vi "Main.vi"() -> ()   [LabVIEW 2015]
uses:
  TypeDefs/FlowData.ctl
  TypeDefs/FluidData.ctl
  TypeDefs/SetFlow.ctl
  TypeDefs/PDCSetup.ctl
  TypeDefs/PDCDisplay.ctl
  TypeDefs/PDCRecordStatus.ctl
  TypeDefs/PDCFrames.ctl
  TypeDefs/PDCSaveSettings.ctl
  TypeDefs/SetRegulation.ctl
  TypeDefs/AutoTrigger.ctl
  TypeDefs/MPXMicropump.ctl
  TypeDefs/PDCLists.ctl
  TypeDefs/ClsLastSample.ctl
  <vilib>/picture/picture.llb/imagedata.ctl
  <vilib>/Utility/xml.llb/Write to XML File(string).vi
  <vilib>/Utility/xml.llb/Read From XML File(string).vi
panel:
  in  "Run Calibration":bool
  in  "Logging Path":path
  in  "FullDropImpact":bool
  in  "MPX Micropump":T1 {"Signal Form" items=["Sinus", "Rechteck", "SRS-Signal"]}
  out "PDCRecordStatus":T2
  out "Standard Deviation of \nFilm Hight over the \nMeasuring Length [µm]":dbl
  in  "ConfigureCls":bool
  out "Film Height [µm]":dbl
  in  "Set Regulation":T3
  out "SaveStatus":i32(slide)=-2046 caption="Downloading Frames from Camera and Saving.... PLEASE WAIT" scale=-200.0..200.0
  out "Picture":picture
  out "Drop Temperature [°C]":dbl
  out "Angle [°]":dbl format="%#.1g"
  in  "Set Flow":T4 {"Set Flow Value" min=0.0 max=100.0}
  out "Fluid Data":T5
  in  "Log Data":bool
  out "Flow Data":T6
  in  "StopALL":bool
  in  "CamTab":enum32{"CamLIVE", "CamSAVE", "PFV"}(tab)
  in  "PDC Setup":T7={"Color Type"=enum."MONO", "Bit Depth"=0, "Resolution"=0, "Record Rate"=0, "Shutter Speed"=0, "Trigger Mode"=0, "Display"=enum."LiveStop"}
  in  "Record":bool caption="Calibrate"
  in  "RecCancel":bool caption="Calibrate"
  in  "SavePDCSetup":bool
  in  "LoadPDCSetup":bool
  in  "Shading":bool
  in  "Auto Trigger":T9={"Auto Trigger"=FALSE, "Sensitivity [0-100]"=98.4} {"Sensitivity [0-100]" min=0.0 max=100.0 format="%.2f"}
  in  "PDCSaveFrames":bool
  in  "PDC Save Settings":T10={"Save Folder"=path "", "File Name"="", "Data Type"=enum."AVI"}
  in  "PDC Frames":T11 {"Current Frame" min=-39378 max=39378; "End Frame" min=-39378 max=39378; "Start Frame" min=-39378 max=39378; "Frames-Slide" scale=-39378.0..39378.0}
  in  "Path of PFV.exe":path=path "C:/Program Files (x86)/Photron/Photron FASTCAM Viewer 3/PFV.exe"
  in  "PDCStartPFV":bool
  # "Auto Triggering Manual:\n1.) Turn ON 'Auto Trigger' BEFORE pressing 'Record' Button\n2.) Press 'Record' Button and wait 4 sec \n3.) Now ready to recognize Drops automatically."
  # "Run PFV to configure cam/save cam data"
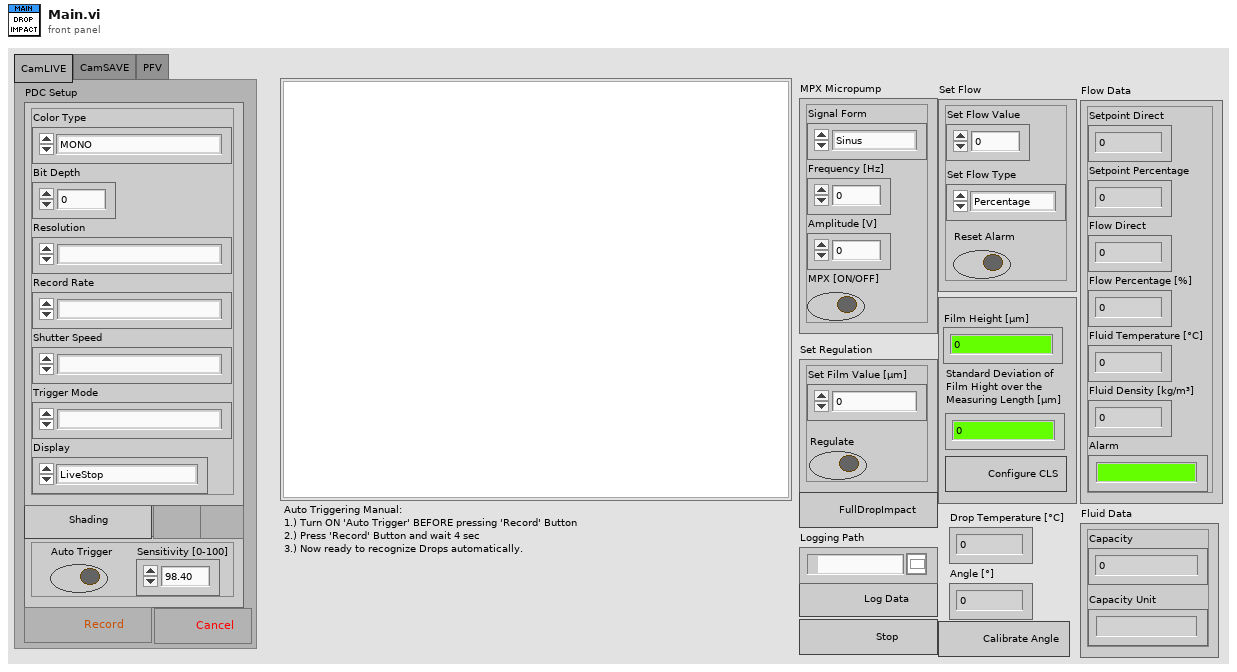
[diagram p1: front panel]
types:
  T1 = typedef "MPXMicropump.ctl" = cluster{"Signal Form":u16, "Frequency [Hz]":i32, "Amplitude [V]":i32, "MPX [ON/OFF]":bool}
  T2 = typedef "PDCRecordStatus.ctl" = enum16{"Live", "Waiting TRG", "Recording"}
  T3 = typedef "SetRegulation.ctl" = cluster{"Set Film Value [µm]":dbl, "Regulate":bool}
  T4 = typedef "SetFlow.ctl" = cluster{"Set Flow Value":dbl, "Set Flow Type":enum16{"Percentage", "Direct"}, "Reset Alarm":bool}
  T5 = typedef "FluidData.ctl" = cluster{"Capacity":sgl, "Capacity Unit":string}
  T6 = typedef "FlowData.ctl" = cluster{"Setpoint Direct":sgl, "Setpoint Percentage":dbl, "Flow Direct":sgl, "Flow Percentage [%]":dbl, "Fluid Temperature [°C]":sgl, "Fluid Density [kg/m³]":sgl, "Alarm":string}
  T7 = typedef "PDCSetup.ctl" = cluster{"Color Type":enum16{"MONO", "COLOR"}, "Bit Depth":i8, "Resolution":u16, "Record Rate":u16, "Shutter Speed":u16, "Trigger Mode":u16, "Display":T8}
  T8 = typedef "PDCDisplay.ctl" = enum16{"Live", "Memory", "LiveStop"}
  T9 = typedef "AutoTrigger.ctl" = cluster{"Auto Trigger":bool, "Sensitivity [0-100]":dbl}
  T10 = typedef "PDCSaveSettings.ctl" = cluster{"Save Folder":path, "File Name":string, "Data Type":enum16{"BMP", "AVI", "MRAW"}}
  T11 = typedef "PDCFrames.ctl" = cluster{"Frames-Slide":i32, "Start Frame":i32, "End Frame":i32, "Current Frame":i32, "PlayFrames":bool}
  T12 = typedef "CommunicationRefs.ctl" = cluster{"ErrorEvent":refnum<user-event>, "DataDisplay":refnum<queue>, "DAQmxAcq":refnum<queue>, "CoriFlow":refnum<queue>, "PrecitecCLS":refnum<queue>, "BartelsMPX":refnum<queue>, "PhotronPDC":refnum<queue>, "JW24F14":refnum<queue>, "Regulator":refnum<queue>, "Logging":refnum<queue>}
  T13 = typedef "ClsLastSample.ctl" = cluster{"Global Signals":dbl[], "Peak Signals":dbl[][], "Film Height [µm]":dbl, "standard deviation [µm]":dbl, "variance":dbl}
  T14 = typedef "PDCLists.ctl" = cluster{"ResolutionList":string[], "RecordRateList":string[], "ShutterSpeedList":string[], "TriggerModeList":string[]}
  T15 = enum8{"Enabled", "Disabled", "Disabled and Grayed Out"}
  T16 = typedef "LVBoundsTypeDef.ctl" = cluster{"Width":u32, "Height":u32}
  T17 = typedef "imagedata.ctl" = cluster{"image type":i32, "image depth":i32, "image":u8[], "mask":u8[], "colors":u32[], "Rectangle":cluster{"left":i16, "top":i16, "right":i16, "bottom":i16}}
  T18 = cluster{"Start":i32, "End":i32, "Trigger":i32, "TwoStageLowToHigh":i32, "TwoStageHighToLow":i32, "TwoStageTiming":u32, "Event":i32[], "EventCount":u32, "RecordedFrames":u32}
  T19 = cluster{"PDC Save Settings":T10, "SaveStatus":refnum<vi>}
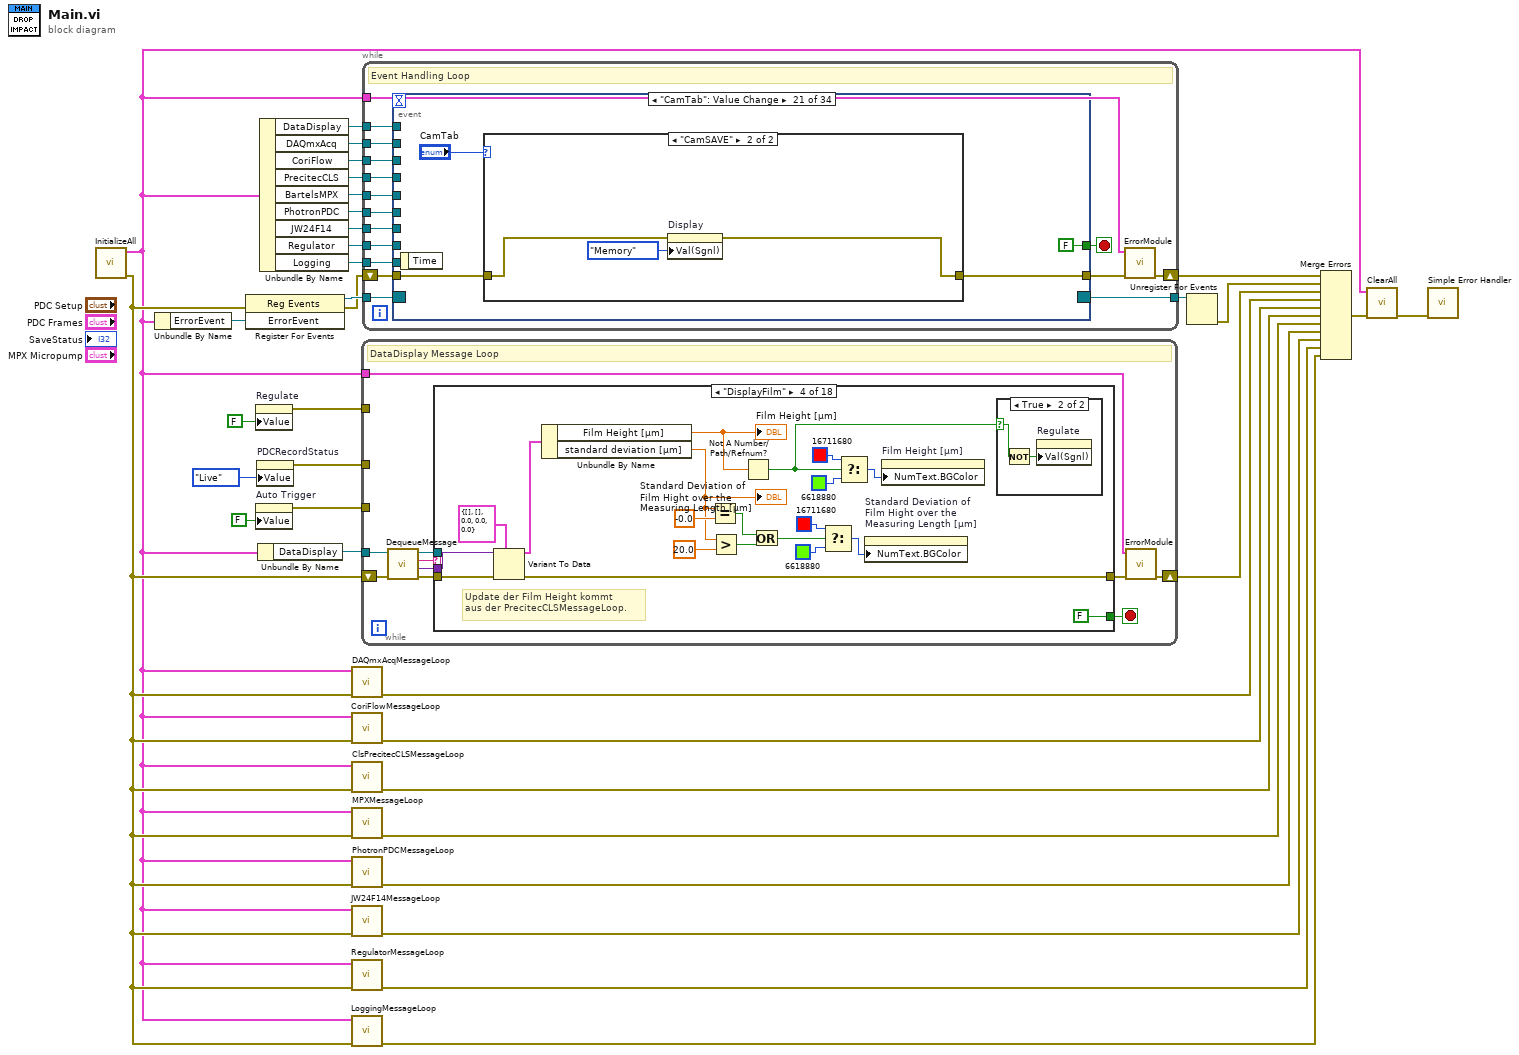
[diagram p0: block diagram]
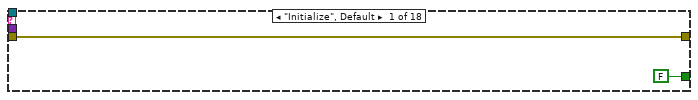
[diagram p2: hidden frame]
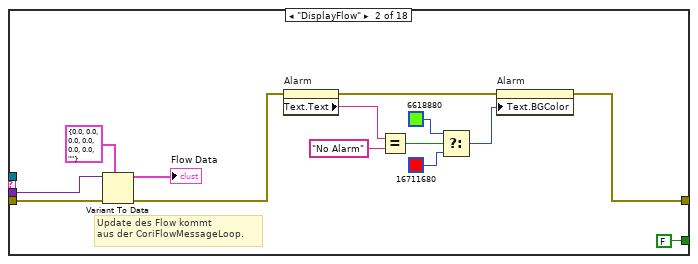
[diagram p3: hidden frame]
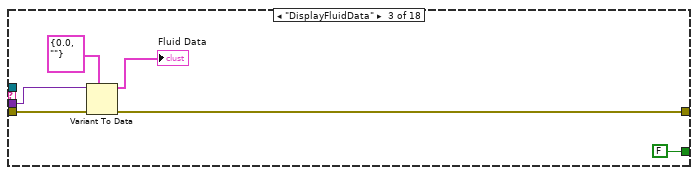
[diagram p4: hidden frame]
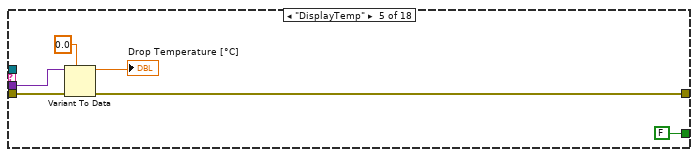
[diagram p6: hidden frame]
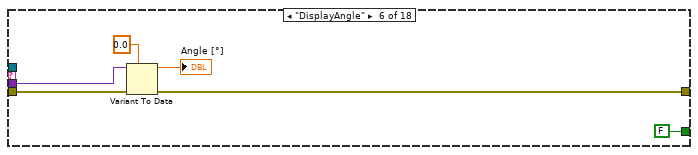
[diagram p7: hidden frame]
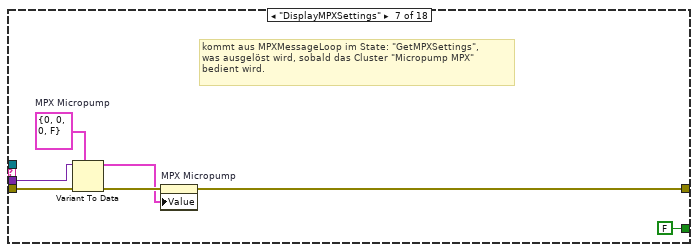
[diagram p8: hidden frame]
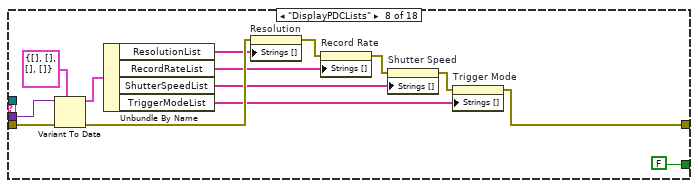
[diagram p9: hidden frame]
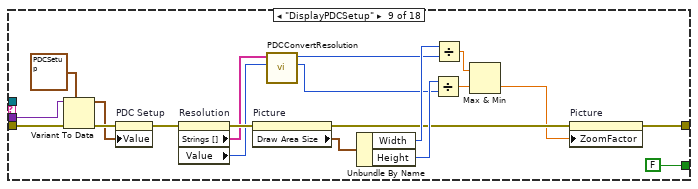
[diagram p10: hidden frame]
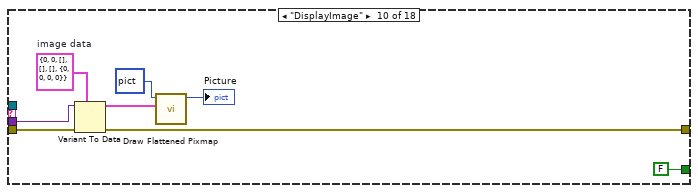
[diagram p11: hidden frame]
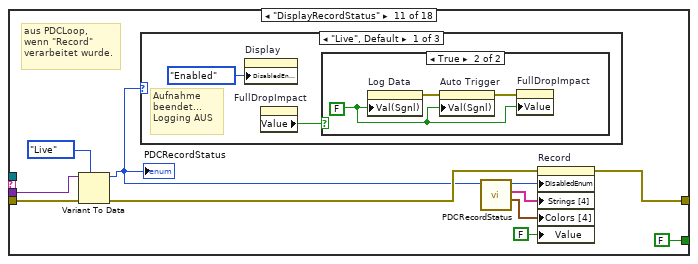
[diagram p12: hidden frame]
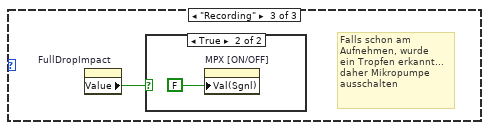
[diagram p15: hidden frame]
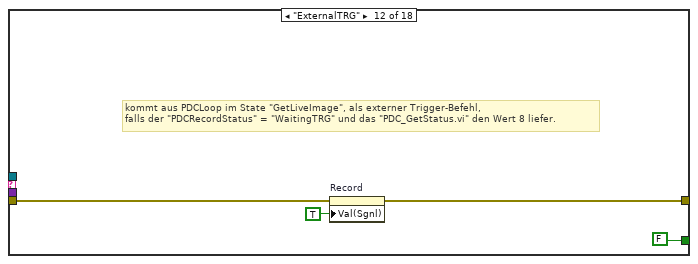
[diagram p17: hidden frame]
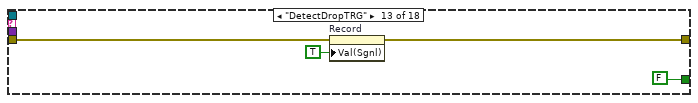
[diagram p18: hidden frame]
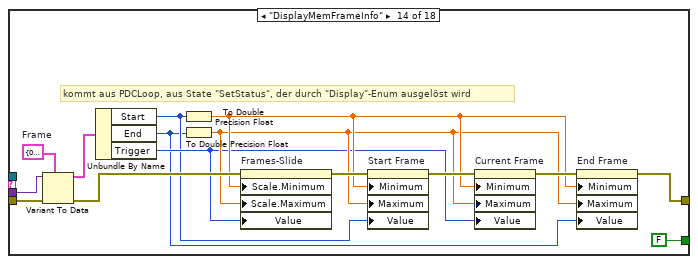
[diagram p19: hidden frame]
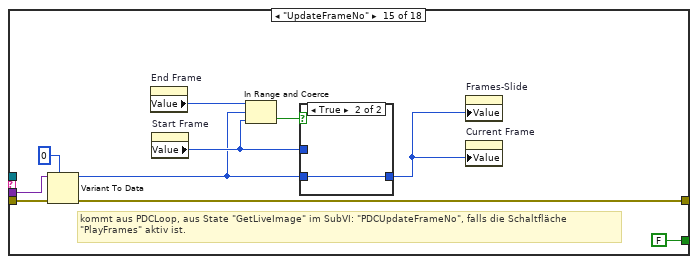
[diagram p20: hidden frame]
diagram:
  n1 = call "InitializeAll.vi"() -> ("Error Out"=w9:errorcluster, "CommunicationRefs"=w1:T12)  [unwired: 10 in]
  n2 = Unbundle By Name(w1) -> ("ErrorEvent"=w30:refnum<user-event>)
  n3 = register-events(error in=w9, w30) -> (reference out=w34:refnum<event-registration>, error out=w31:errorcluster)  [unwired: 1 in]
  n4 = property on="Regulate" class="Bool (strict)"("Value"=FALSE) -> (error out=w2:errorcluster)  [unwired: 2 in, 1 out]
  n5 = property on="Auto Trigger" class="Bool (strict)"("Value"=FALSE) -> (error out=w4:errorcluster)  [unwired: 2 in, 1 out]
  n6 = property on="PDCRecordStatus" class="Enum (strict)"("Value"=PDCRecordStatus."Live" ("PDCRecordStatus")) -> (error out=w12:errorcluster)  [unwired: 2 in, 1 out]
  n7 = Unbundle By Name(w1) -> ("DataDisplay"=w23:refnum<queue>)
  n8 = Unbundle By Name(w1) -> ("DataDisplay"=w21:refnum<queue>, "DAQmxAcq"=w20:refnum<queue>, "CoriFlow"=w19:refnum<queue>, "PrecitecCLS"=w18:refnum<queue>, "BartelsMPX"=w17:refnum<queue>, "PhotronPDC"=w16:refnum<queue>, "JW24F14"=w13:refnum<queue>, "Regulator"=w6:refnum<queue>, "Logging"=w10:refnum<queue>)
  n9 = call "DAQmxAcqMessageLoop.vi"("Error In"=w9, "CommunicationRefs"=w1) -> ("Error Out"=w27:errorcluster)  [unwired: 9 in]
  n10 = call "CoriFlowMessageLoop.vi"("Error In"=w9, "CommunicationRefs"=w1) -> ("Error Out"=w26:errorcluster)  [unwired: 9 in]
  n11 = call "ClsPrecitecCLSMessageLoop.vi"("Error In"=w9, "CommunicationRefs"=w1) -> ("Error Out"=w25:errorcluster)  [unwired: 9 in]
  n12 = call "MPXMessageLoop.vi"("Error In"=w9, "CommunicationRefs"=w1) -> ("Error Out"=w24:errorcluster)  [unwired: 9 in]
  n13 = call "PhotronPDCMessageLoop.vi"("Error In"=w9, "CommunicationRefs"=w1) -> ("Error Out"=w15:errorcluster)  [unwired: 9 in]
  n14 = call "JW24F14MessageLoop.vi"("Error In"=w9, "CommunicationRefs"=w1) -> ("Error Out"=w14:errorcluster)  [unwired: 9 in]
  n15 = call "RegulatorMessageLoop.vi"("Error In"=w9, "CommunicationRefs"=w1) -> ("Error Out"=w8:errorcluster)  [unwired: 9 in]
  n16 = call "LoggingMessageLoop.vi"("Error In"=w9, "CommunicationRefs"=w1) -> ("Error Out"=w7:errorcluster)  [unwired: 9 in]
  n17 = while {
    tunnel: w23 -> [w45]
    tunnel: w1 -> [w38]
    shift-right: [w39] -> w22
    shift-left: w9 -> [w44]
    tunnel: w12 -> [_]
    tunnel: w4 -> [_]
    tunnel: w2 -> [_]
    stop <- w37 stop-if-true
    # "DataDisplay Message Loop"
    n18 = call "DequeueMessage.vi"("error in (no error)"=w44, "MessageQueue"=w45) -> ("error out"=w40:errorcluster, "MessageData"=w41:variant, "Message"=w42:string, "dupMessageQueue"=w43:refnum<queue>)  [unwired: 6 in]
    n19 = case shown="\"DisplayFilm\"" w42 {
      tunnel: w43 -> [_ _ _ _ _ _ _ _ _ _ _ _ _ _ _ _ _ _]
      tunnel: w41 -> [_ w61 w65 w85 w94 w99 w107 w120 w140 w148 w158 _ _ w190 w199 _ _ _]
      tunnel: w40 -> [w46 w60 w67 w86 w91 w98 w108 w121 w142 w150 w160 w172 w174 w191 w200 w206 w210 w219]
      tunnel: [w46 w49 w66 w76 w90 w97 w104 w109 w129 w147 w151 w171 w173 w182 w197 w204 w208 w219] -> w36
      tunnel: [FALSE FALSE FALSE FALSE FALSE FALSE FALSE FALSE FALSE FALSE FALSE FALSE FALSE FALSE FALSE FALSE FALSE TRUE] -> w37
      frame "Initialize", Default {
      }
      frame "DisplayFlow" {
        # "Update des Flow kommt \naus der CoriFlowMessageLoop."
        n20 = Variant To Data(error in=w60, type=T6 {"Setpoint Direct"=0.0, "Setpoint Percentage"=0.0, "Flow Direct"=0.0, "Flow Percentage [%]"=0.0, "Fluid Temperature [°C]"=0.0, "Fluid Density [kg/m³]"=0.0, "Alarm"=""} ("Sensor Data"), Variant=w61) -> (data=→"Flow Data":T6, error out=w52:errorcluster)
        n21 = property on="Alarm" class="Str"(error in=w52) -> (error out=w50:errorcluster, "Text.Text"=w51:string)  [unwired: 1 in, 1 out]
        n22 = Equal?(x=w51, y="No Alarm") -> (x = y?=w56:bool)
        n23 = Select(t=u32 6618880, s=w56, f=u32 16711680) -> (s? t:f=w48:u32)
        n24 = property on="Alarm" class="Str"(error in=w50, "Text.BGColor"=w48) -> (error out=w49:errorcluster)  [unwired: 1 in, 1 out]
      }
      frame "DisplayFluidData" {
        n25 = Variant To Data(error in=w67, type=T5 {"Capacity"=0.0, "Capacity Unit"=""} ("Fluid Data"), Variant=w65) -> (data=→"Fluid Data":T5, error out=w66:errorcluster)
      }
      frame "DisplayFilm" {
        # "Update der Film Height kommt \naus der PrecitecCLSMessageLoop."
        n26 = Variant To Data(error in=w86, type=T13 {"Global Signals"=[], "Peak Signals"=[], "Film Height [µm]"=0.0, "standard deviation [µm]"=0.0, "variance"=0.0} ("ClsLastSample"), Variant=w85) -> (data=w83:T13, error out=w76:errorcluster)
        n27 = Unbundle By Name(w83) -> ("Film Height [µm]"=w82:dbl, "standard deviation [µm]"=w78:dbl)
        "Film Height [µm]" <- w82
        "Standard Deviation of \nFilm Hight over the \nMeasuring Length [µm]" <- w78
        n28 = Equal?(x=w78, y=-0.0) -> (x = y?=w80:bool)
        n29 = Greater?(x=w78, y=20.0) -> (0:w79:bool)
        n30 = Not A Number/Path/Refnum?(number/path/refnum=w82) -> (NaN/Path/Refnum?=w68:bool)
        n31 = Or(x=w80, y=w79) -> (x .or. y?=w73:bool)
        n32 = Select(t=u32 16711680, s=w73, f=u32 6618880) -> (s? t:f=w72:u32)
        n33 = Select(t=u32 16711680, s=w68, f=u32 6618880) -> (s? t:f=w69:u32)
        n34 = property on="Standard Deviation of \nFilm Hight over the \nMeasuring Length [µm]" class="DigNum (strict)"("NumText.BGColor"=w72) -> ()  [unwired: 2 in, 2 out]
        n35 = property on="Film Height [µm]" class="DigNum (strict)"("NumText.BGColor"=w69) -> ()  [unwired: 2 in, 2 out]
        n36 = case shown="True" w68 {
          selector: w68 -> [_ w89]
          frame False {
          }
          frame True {
            n37 = Not(x=w89) -> (.not. x?=w88:bool)
            n38 = property on="Regulate" class="Bool (strict)"("Val(Sgnl)"=w88) -> ()  [unwired: 2 in, 2 out]
          }
        }
      }
      frame "DisplayTemp" {
        n39 = Variant To Data(error in=w91, type=0.0, Variant=w94) -> (data=→"Drop Temperature [°C]":dbl, error out=w90:errorcluster)
      }
      frame "DisplayAngle" {
        n40 = Variant To Data(error in=w98, type=0.0, Variant=w99) -> (data=→"Angle [°]":dbl, error out=w97:errorcluster)
      }
      frame "DisplayMPXSettings" {
        w103 = T1 {"Signal Form"=0, "Frequency [Hz]"=0, "Amplitude [V]"=0, "MPX [ON/OFF]"=FALSE}  # MPX Micropump
        # "kommt aus MPXMessageLoop im State: \"GetMPXSettings\",\nwas ausgelöst wird, sobald das Cluster \"Micropump MPX\"\nbedient wird."
        n41 = Variant To Data(error in=w108, type=w103, Variant=w107) -> (data=w102:T1, error out=w105:errorcluster)
        n42 = property on="MPX Micropump" class="Clust (strict)"(error in=w105, "Value"=w102) -> (error out=w104:errorcluster)  [unwired: 1 in, 1 out]
      }
      frame "DisplayPDCLists" {
        n43 = Variant To Data(error in=w121, type=T14 {"ResolutionList"=[], "RecordRateList"=[], "ShutterSpeedList"=[], "TriggerModeList"=[]} ("PDCLists"), Variant=w120) -> (data=w117:T14, error out=w122:errorcluster)
        n44 = Unbundle By Name(w117) -> ("ResolutionList"=w116:string[], "RecordRateList"=w115:string[], "ShutterSpeedList"=w113:string[], "TriggerModeList"=w110:string[])
        n45 = property on="Resolution" class="Ring (strict)"(error in=w122, "Strings []"=w116) -> (error out=w114:errorcluster)  [unwired: 1 in, 1 out]
        n46 = property on="Record Rate" class="Ring (strict)"(error in=w114, "Strings []"=w115) -> (error out=w112:errorcluster)  [unwired: 1 in, 1 out]
        n47 = property on="Shutter Speed" class="Ring (strict)"(error in=w112, "Strings []"=w113) -> (error out=w111:errorcluster)  [unwired: 1 in, 1 out]
        n48 = property on="Trigger Mode" class="Ring (strict)"(error in=w111, "Strings []"=w110) -> (error out=w109:errorcluster)  [unwired: 1 in, 1 out]
      }
      frame "DisplayPDCSetup" {
        n49 = Variant To Data(error in=w142, type=T7 {"Color Type"=enum."MONO", "Bit Depth"=0, "Resolution"=0, "Record Rate"=0, "Shutter Speed"=0, "Trigger Mode"=0, "Display"=enum."LiveStop"} ("PDC Setup"), Variant=w140) -> (data=w137:T7, error out=w138:errorcluster)
        n50 = property on="PDC Setup" class="Clust (strict)"(error in=w138, "Value"=w137) -> (error out=w132:errorcluster)  [unwired: 1 in, 1 out]
        n51 = property on="Resolution" class="Ring (strict)"(error in=w132) -> (error out=w131:errorcluster, "Strings []"=w127:string[], "Value"=w126:u16)  [unwired: 1 in, 1 out]
        n52 = property on="Picture" class="Pict"(error in=w131) -> (error out=w128:errorcluster, "Draw Area Size"=w130:T16)  [unwired: 1 in, 1 out]
        n53 = call "PDCConvertResolution.vi"("ResValue"=w126, "ResStrings"=w127) -> ("Height"=w124:u32, "Width"=w125:u32)  [unwired: 8 in]
        n54 = Unbundle By Name(w130) -> ("Width"=w133:u32, "Height"=w134:u32)
        n55 = Divide(x=w134, y=w124) -> (x/y=w136:dbl)
        n56 = Divide(x=w133, y=w125) -> (x/y=w135:dbl)
        n57 = Max & Min(x=w135, y=w136) -> (min(x,y)=w123:dbl)  [unwired: 1 out]
        n58 = property on="Picture" class="Pict"(error in=w128, "ZoomFactor"=w123) -> (error out=w129:errorcluster)  [unwired: 1 in, 1 out]
      }
      frame "DisplayImage" {
        w146 = T17 {"image type"=0, "image depth"=0, "image"=[], "mask"=[], "colors"=[], "Rectangle"={"left"=0, "top"=0, "right"=0, "bottom"=0}}  # image data
        n59 = Variant To Data(error in=w150, type=w146, Variant=w148) -> (data=w145:T17, error out=w147:errorcluster)
        n60 = call <vilib>:"Draw Flattened Pixmap.vi"("image data"=w145, "picture"=picture data[5B]) -> ("new picture"=→"Picture":picture)  [unwired: 7 in]
      }
      frame "DisplayRecordStatus" {
        # "aus PDCLoop, \nwenn \"Record\" \nverarbeitet wurde."
        n61 = Variant To Data(error in=w160, type=PDCRecordStatus."Live" ("PDCRecordStatus"), Variant=w158) -> (data=w152:T2, error out=w161:errorcluster)
        "PDCRecordStatus" <- w152
        n62 = case shown="\"Live\", Default" w152 {
          frame "Live", Default {
            # "Aufnahme\nbeendet...\nLogging AUS"
            n63 = property on="Display" class="Enum (strict)"("DisabledEnum"=T15."Enabled" ("Disabled")) -> ()  [unwired: 2 in, 2 out]
            n64 = property on="FullDropImpact" class="Bool (strict)"() -> ("Value"=w162:bool)  [unwired: 2 in, 2 out]
            n65 = case shown="True" w162 {
              frame False {
              }
              frame True {
                w164 = FALSE ("Value (Signaling)")
                n66 = property on="Log Data" class="Bool (strict)"("Val(Sgnl)"=w164) -> (error out=w166:errorcluster)  [unwired: 2 in, 1 out]
                n67 = property on="Auto Trigger" class="Bool (strict)"(error in=w166, "Val(Sgnl)"=w164) -> (error out=w165:errorcluster)  [unwired: 1 in, 1 out]
                n68 = property on="FullDropImpact" class="Bool (strict)"(error in=w165, "Value"=w164) -> ()  [unwired: 1 in, 2 out]
              }
            }
          }
          frame "Waiting TRG" {
          }
          frame "Recording" {
            # "Falls schon am \nAufnehmen, wurde\nein Tropfen erkannt...\ndaher Mikropumpe \nausschalten"
            n69 = property on="FullDropImpact" class="Bool (strict)"() -> ("Value"=w167:bool)  [unwired: 2 in, 2 out]
            n70 = case shown="True" w167 {
              frame False {
              }
              frame True {
                n71 = property on="MPX [ON/OFF]" class="Bool (strict)"("Val(Sgnl)"=FALSE ("Value (Signaling)")) -> ()  [unwired: 2 in, 2 out]
              }
            }
          }
        }
        n72 = call "PDCRecordStatus.vi"("PDCRecordStatus"=w152) -> ("Color[4]"=w154:cluster{u32, u32}[], "String[4]"=w156:string[], "Disabled"=w155:T15)  [unwired: 8 in]
        n73 = property on="Record" class="Bool (strict)"(error in=w161, "DisabledEnum"=w155, "Strings [4]"=w156, "Colors [4]"=w154, "Value"=FALSE ("Record")) -> (error out=w151:errorcluster)  [unwired: 1 in, 1 out]
      }
      frame "ExternalTRG" {
        # "kommt aus PDCLoop im State \"GetLiveImage\", als externer Trigger-Befehl,\nfalls der \"PDCRecordStatus\" = \"WaitingTRG\" und das \"PDC_GetStatus.vi\" den Wert 8 liefer."
        n74 = property on="Record" class="Bool (strict)"(error in=w172, "Val(Sgnl)"=TRUE ("Value (Signaling)")) -> (error out=w171:errorcluster)  [unwired: 1 in, 1 out]
      }
      frame "DetectDropTRG" {
        n75 = property on="Record" class="Bool (strict)"(error in=w174, "Val(Sgnl)"=TRUE ("Value (Signaling)")) -> (error out=w173:errorcluster)  [unwired: 1 in, 1 out]
      }
      frame "DisplayMemFrameInfo" {
        w189 = T18 {"Start"=0, "End"=0, "Trigger"=0, "TwoStageLowToHigh"=0, "TwoStageHighToLow"=0, "TwoStageTiming"=0, "Event"=[1, 1, 1, 1, 1, 1, 1, 1, 1, 1], "EventCount"=0, "RecordedFrames"=0}  # Frame
        # "kommt aus PDCLoop, aus State \"SetStatus\", der durch \"Display\"-Enum ausgelöst wird"
        n76 = Variant To Data(error in=w191, type=w189, Variant=w190) -> (data=w188:T18, error out=w186:errorcluster)
        n77 = Unbundle By Name(w188) -> ("Start"=w178:i32, "End"=w177:i32, "Trigger"=w179:i32)
        n78 = To Double Precision Float(number=w178) -> (double precision float=w181:dbl)
        n79 = To Double Precision Float(number=w177) -> (double precision float=w180:dbl)
        n80 = property on="Frames-Slide" class="Slide (strict)"(error in=w186, "Scale.Minimum"=w181, "Scale.Maximum"=w180, "Value"=w179) -> (error out=w185:errorcluster)  [unwired: 1 in, 1 out]
        n81 = property on="Start Frame" class="DigNum (strict)"(error in=w185, "Minimum"=w181, "Maximum"=w180, "Value"=w178) -> (error out=w184:errorcluster)  [unwired: 1 in, 1 out]
        n82 = property on="Current Frame" class="DigNum (strict)"(error in=w184, "Minimum"=w181, "Maximum"=w180, "Value"=w179) -> (error out=w183:errorcluster)  [unwired: 1 in, 1 out]
        n83 = property on="End Frame" class="DigNum (strict)"(error in=w183, "Minimum"=w181, "Maximum"=w180, "Value"=w177) -> (error out=w182:errorcluster)  [unwired: 1 in, 1 out]
      }
      frame "UpdateFrameNo" {
        # "kommt aus PDCLoop, aus State \"GetLiveImage\" im SubVI: \"PDCUpdateFrameNo\", falls die Schaltfläche\n\"PlayFrames\" aktiv ist."
        n84 = Variant To Data(error in=w200, type=0 ("Value (Signaling)"), Variant=w199) -> (data=w192:i32, error out=w197:errorcluster)
        n85 = property on="End Frame" class="DigNum (strict)"() -> ("Value"=w193:i32)  [unwired: 2 in, 2 out]
        n86 = property on="Start Frame" class="DigNum (strict)"() -> ("Value"=w195:i32)  [unwired: 2 in, 2 out]
        n87 = In Range and Coerce(upper limit=w193, x=w192, lower limit=w195) -> (In Range?=w194:bool)  [unwired: 1 out]
        n88 = case shown="True" w194 {
          tunnel: w195 -> [w202 _]
          tunnel: w192 -> [_ w203]
          tunnel: [w202 w203] -> w196
          frame False {
          }
          frame True {
          }
        }
        n89 = property on="Frames-Slide" class="Slide (strict)"("Value"=w196) -> ()  [unwired: 2 in, 2 out]
        n90 = property on="Current Frame" class="DigNum (strict)"("Value"=w196) -> ()  [unwired: 2 in, 2 out]
      }
      frame "PDCDataSaveFinished" {
        # "kommt aus PDCLoop, aus State \"PDCDataSave\", wenn das Abspeichern der Frames abgeschlossen ist."
        n91 = property on="CamTab" class="TabCtl (strict)"(error in=w206, "DisabledEnum"=T15."Enabled" ("Disabled")) -> (error out=w204:errorcluster)  [unwired: 1 in, 1 out]
      }
      frame "RefImageTaken" {
        n92 = property on="FullDropImpact" class="Bool (strict)"(error in=w210) -> (error out=w209:errorcluster, "Value"=w211:bool)  [unwired: 1 in, 1 out]
        n93 = case shown="True" w211 {
          tunnel: w209 -> [w213 w215]
          tunnel: [w213 w214] -> w208
          frame False {
          }
          frame True {
            w216 = TRUE ("Value (Signaling)")
            n94 = property on="MPX [ON/OFF]" class="Bool (strict)"(error in=w215, "Val(Sgnl)"=w216) -> (error out=w217:errorcluster)  [unwired: 1 in, 1 out]
            n95 = property on="Log Data" class="Bool (strict)"(error in=w217, "Val(Sgnl)"=w216) -> (error out=w214:errorcluster)  [unwired: 1 in, 1 out]
          }
        }
      }
      frame "Stop" {
      }
    }
    n96 = call "ErrorModule.vi"("Error In"=w36, "CommunicationRefs"=w38) -> ("Error Out"=w39:errorcluster)  [unwired: 9 in]
  }
  n97 = while {
    tunnel: w34 -> [w235]
    tunnel: [w233] -> w33
    shift-right: [w231] -> w29
    shift-left: w31 -> [w232]
    tunnel: w1 -> [w229]
    tunnel: w20 -> [w228]
    tunnel: w19 -> [w227]
    tunnel: w18 -> [w226]
    tunnel: w17 -> [w225]
    tunnel: w6 -> [w224]
    tunnel: w21 -> [w223]
    tunnel: w16 -> [w222]
    tunnel: w13 -> [w221]
    tunnel: w10 -> [w220]
    stop <- w234 stop-if-true
    # "Event Handling Loop"
    n98 = event shown="[20] \"CamTab\": Value Change" {
      selector: w235 -> [_ _ _ _ _ _ _ _ _ _ _ _ _ _ _ _ _ _ _ _ _ _ _ _ _ _ _ _ _ _ _ _ _ _]
      dyn-events: [_ _ _ _ _ _ _ _ _ _ _ _ _ _ _ _ _ _ _ _ _ _ _ _ _ _ _ _ _ _ _ _ _ _] -> w233
      timeout: _ -> [_ _ _ _ _ _ _ _ _ _ _ _ _ _ _ _ _ _ _ _ _ _ _ _ _ _ _ _ _ _ _ _ _ _]
      tunnel: ["StopALL" w252 FALSE ("Error") FALSE ("Error") FALSE ("Error") FALSE ("Error") FALSE ("Error") FALSE ("Error") FALSE ("Error") FALSE ("Error") FALSE ("Error") FALSE ("Error") FALSE ("Error") FALSE ("Error") FALSE ("Error") FALSE ("Error") FALSE ("Error") FALSE ("Error") FALSE ("Error") FALSE ("Error") FALSE ("Error") FALSE ("Error") FALSE ("Error") FALSE ("Error") FALSE ("Error") FALSE ("Error") FALSE ("Error") FALSE ("Error") FALSE ("Error") FALSE ("Error") FALSE ("Error") FALSE ("Error") FALSE ("Error") FALSE ("Error")] -> w234
      tunnel: [w247 w251 w263 w288 w301 w306 w313 w337 w344 w351 w358 w365 w372 w375 w393 w402 w405 w414 w429 w432 w441 w452 w459 w483 w507 w522 w532 w552 w568 w592 w598 w615 w646 w681] -> w230
      tunnel: w232 -> [w247 w251 w264 w284 w302 w307 w314 w338 w345 w352 w359 w366 w373 w376 w394 w403 w412 w419 w423 w436 w442 w455 w456 w480 w513 w523 w524 w553 w570 w593 w599 w616 w645 w682]
      tunnel: w228 -> [w245 _ w261 _ _ _ _ _ _ _ _ _ _ _ _ _ _ _ _ _ _ _ _ _ _ _ _ _ _ _ _ _ _ _]
      tunnel: w227 -> [w244 _ w260 w293 w303 _ _ _ _ _ _ _ _ _ _ _ _ _ _ _ _ _ _ _ _ _ _ _ _ _ _ _ _ _]
      tunnel: w226 -> [w243 _ w259 _ _ _ _ _ _ _ _ _ _ _ _ _ _ _ _ _ _ _ _ _ _ _ _ _ _ _ _ _ _ w684]
      tunnel: w225 -> [w242 _ w258 _ _ _ _ w339 w346 w353 w360 _ _ _ _ _ _ _ _ _ _ _ _ _ _ _ _ _ _ _ _ _ _ _]
      tunnel: w224 -> [w237 _ _ _ _ w311 _ _ _ _ _ _ _ _ _ _ _ _ _ _ _ _ _ _ _ _ _ _ _ _ _ _ _ _]
      tunnel: w223 -> [w241 _ _ _ _ _ _ _ _ _ _ _ _ _ _ _ _ _ _ _ _ _ _ _ _ _ _ _ _ _ _ _ _ _]
      tunnel: w222 -> [w239 _ w255 _ _ _ _ _ _ _ _ w367 w374 w386 w395 w404 w413 w420 w428 w438 _ _ w457 w481 w506 w520 w530 _ w567 w590 w596 w611 _ _]
      tunnel: w221 -> [w238 _ w254 _ _ _ _ _ _ _ _ _ _ _ _ _ _ _ _ _ _ _ _ _ _ _ _ _ _ _ _ _ w644 _]
      tunnel: w220 -> [w236 _ w253 _ _ _ _ _ _ _ _ _ _ _ _ _ _ _ _ _ _ _ _ _ _ _ _ _ _ _ _ _ _ _]
      event "StopALL": Value Change; Panel Close {
        # "Stoppt die Event-Schleife und sendet eine Nachricht \nan alle anderen Schleifen zum Stoppen."
        n99 = event-data() -> ()  [unwired: 1 in, 1 out]
        n100 = Build Array(w241, w245, w244, w243, w242, w239, w238, w237, w236) -> (w240:refnum<queue>[])
        n101 = for {
          tunnel: w240 -> [w250] mode=indexing
          workers-P: _ -> [_]
          n102 = call "EnqueueMessage.vi"("Priority Message? (F)"=TRUE, "Message"="Stop", "MessageQueue"=w250) -> ()  [unwired: 7 in, 2 out]
        }
      }
      event User Event {
        # "Das ErrorEvent wird ausgelöst, falls in einer der Schleifen ein Error\ndurch das Error-Modul festgestellt wird... und dient zum\nStoppen der Event-Schleife"
        n103 = event-data() -> ("Error"=w252:bool)  [unwired: 1 in]
      }
      event "Log Data": Value Change {
        n104 = event-data() -> ()  [unwired: 1 in, 1 out]
        n105 = Build Array(w261, w260, w259, w258, w255, w254, w253) -> (w257:refnum<queue>[])
        n106 = for {
          tunnel: "Log Data" -> [w266]
          shift-right: [w267] -> w263
          shift-left: w264 -> [w268]
          tunnel: w257 -> [w265] mode=indexing
          n107 = case shown="True" w266 {
            tunnel: w265 -> [w275 w280]
            tunnel: w268 -> [w273 w278]
            tunnel: [w272 w277] -> w267
            frame True {
              n108 = To Variant(anything="Logging Path") -> (Variant=w269:variant)
              n109 = call "EnqueueMessage.vi"("Priority Message? (F)"=TRUE, "error in (no error)"=w273, "MessageData"=w269, "Message"="StartLogging", "MessageQueue"=w275) -> ("error out"=w272:errorcluster)  [unwired: 5 in, 1 out]
            }
            frame False {
              n110 = call "EnqueueMessage.vi"("Priority Message? (F)"=TRUE, "error in (no error)"=w278, "Message"="StopLogging", "MessageQueue"=w280) -> ("error out"=w277:errorcluster)  [unwired: 6 in, 1 out]
            }
          }
        }
      }
      event Value Change {
        n111 = event-data() -> ()  [unwired: 1 in, 1 out]
        n112 = property on="Set Flow Type" class="Enum (strict)"(error in=w284) -> (error out=w283:errorcluster, "Value"=w287:enum16{"Percentage", "Direct"})  [unwired: 1 in, 1 out]
        n113 = case shown="\"Percentage\", Default" w287 {
          tunnel: [sgl 100.0 ("Value") w298] -> w286
          tunnel: w283 -> [w294 w297]
          tunnel: [w294 w296] -> w282
          frame "Percentage", Default {
          }
          frame "Direct" {
            n114 = property on="Capacity" class="DigNum (strict)"(error in=w297) -> (error out=w296:errorcluster, "Value"=w298:sgl)  [unwired: 1 in, 1 out]
          }
        }
        n115 = property on="Set Flow Value" class="DigNum (strict)"(error in=w282, "Maximum"=w286, "Minimum"=0.0 ("Data Entry Limits:Minimum")) -> (error out=w281:errorcluster)  [unwired: 1 in, 1 out]
        n116 = To Variant(anything="Set Flow") -> (Variant=w291:variant)
        n117 = call "EnqueueMessage.vi"("error in (no error)"=w281, "MessageData"=w291, "Message"="SetFlow", "MessageQueue"=w293) -> ("error out"=w288:errorcluster)  [unwired: 6 in, 1 out]
      }
      event Value Change {
        n118 = event-data() -> ()  [unwired: 1 in, 1 out]
        n119 = call "EnqueueMessage.vi"("error in (no error)"=w302, "Message"="ResetAlarm", "MessageQueue"=w303) -> ("error out"=w301:errorcluster)  [unwired: 7 in, 1 out]
      }
      event Value Change {
        n120 = event-data() -> ()  [unwired: 1 in, 1 out]
        n121 = To Variant(anything="Set Regulation") -> (Variant=w310:variant)
        n122 = call "EnqueueMessage.vi"("Priority Message? (F)"=TRUE, "error in (no error)"=w307, "MessageData"=w310, "Message"="SetRegulation", "MessageQueue"=w311) -> ("error out"=w306:errorcluster)  [unwired: 5 in, 1 out]
      }
      event "FullDropImpact": Value Change {
        n123 = event-data() -> ()  [unwired: 1 in, 1 out]
        n124 = case shown="True" "FullDropImpact" {
          tunnel: w314 -> [w316 w319]
          tunnel: [w316 w321] -> w313
          frame False {
          }
          frame True {
            n125 = call "File Dialog3"("pattern (all files)"="*.tdms") -> ("selected path"=w318:path)  [unwired: 11 in, 3 out]
            n126 = call <vilib>:"Is Path and Not Empty.vi"("path"=w318) -> ("Is Path and Not Empty?"=w317:bool)  [unwired: 4 in]
            n127 = case shown="True" w317 {
              tunnel: [w324 w330] -> w321
              tunnel: w318 -> [_ w327]
              tunnel: w319 -> [w324 w326]
              frame False {
                n128 = property on="FullDropImpact" class="Bool (strict)"("Value"=FALSE ("FullDropImpact")) -> ()  [unwired: 2 in, 2 out]
                n129 = One Button Dialog(message="INVALID \"Logging Path\".") -> ()  [unwired: 1 in, 1 out]
              }
              frame True {
                w331 = TRUE ("Value (Signaling)")
                n130 = property on="Logging Path" class="Path"(error in=w326, "Value"=w327) -> (error out=w325:errorcluster)  [unwired: 1 in, 1 out]
                n131 = property on="Regulate" class="Bool (strict)"(error in=w325, "Val(Sgnl)"=FALSE ("Value (Signaling)")) -> (error out=w329:errorcluster)  [unwired: 1 in, 1 out]
                n132 = property on="Auto Trigger" class="Bool (strict)"(error in=w329, "Val(Sgnl)"=w331) -> (error out=w332:errorcluster)  [unwired: 1 in, 1 out]
                n133 = property on="Record" class="Bool (strict)"(error in=w332, "Val(Sgnl)"=w331) -> (error out=w330:errorcluster)  [unwired: 1 in, 1 out]
              }
            }
          }
        }
      }
      event Value Change {
        n134 = event-data() -> ("NewVal"=w333:bool)  [unwired: 1 in]
        n135 = To Variant(anything=w333) -> (Variant=w334:variant)
        n136 = call "EnqueueMessage.vi"("error in (no error)"=w338, "MessageData"=w334, "Message"="SetOnOff", "MessageQueue"=w339) -> ("error out"=w337:errorcluster)  [unwired: 6 in, 1 out]
      }
      event Value Change {
        n137 = event-data() -> ("NewVal"=w340:u16)  [unwired: 1 in]
        n138 = To Variant(anything=w340) -> (Variant=w341:variant)
        n139 = call "EnqueueMessage.vi"("error in (no error)"=w345, "MessageData"=w341, "Message"="SetSignalForm", "MessageQueue"=w346) -> ("error out"=w344:errorcluster)  [unwired: 6 in, 1 out]
      }
      event Value Change {
        n140 = event-data() -> ("NewVal"=w347:i32)  [unwired: 1 in]
        n141 = To Variant(anything=w347) -> (Variant=w348:variant)
        n142 = call "EnqueueMessage.vi"("error in (no error)"=w352, "MessageData"=w348, "Message"="SetFrequency", "MessageQueue"=w353) -> ("error out"=w351:errorcluster)  [unwired: 6 in, 1 out]
      }
      event Value Change {
        n143 = event-data() -> ("NewVal"=w354:i32)  [unwired: 1 in]
        n144 = To Variant(anything=w354) -> (Variant=w355:variant)
        n145 = call "EnqueueMessage.vi"("error in (no error)"=w359, "MessageData"=w355, "Message"="SetAmplitude", "MessageQueue"=w360) -> ("error out"=w358:errorcluster)  [unwired: 6 in, 1 out]
      }
      event Value Change {
        n146 = event-data() -> ("NewVal"=w361:enum16{"MONO", "COLOR"})  [unwired: 1 in]
        n147 = To Variant(anything=w361) -> (Variant=w362:variant)
        n148 = call "EnqueueMessage.vi"("error in (no error)"=w366, "MessageData"=w362, "Message"="SetColorType", "MessageQueue"=w367) -> ("error out"=w365:errorcluster)  [unwired: 6 in, 1 out]
      }
      event Value Change {
        n149 = event-data() -> ("NewVal"=w368:i8)  [unwired: 1 in]
        n150 = To Variant(anything=w368) -> (Variant=w369:variant)
        n151 = call "EnqueueMessage.vi"("error in (no error)"=w373, "MessageData"=w369, "Message"="SetBitDepth", "MessageQueue"=w374) -> ("error out"=w372:errorcluster)  [unwired: 6 in, 1 out]
      }
      event Value Change {
        w377 = cluster{"Width":u32, "Height":u32} {"Width"=0, "Height"=0}  # Resolution
        n152 = event-data() -> ("NewVal"=w381:u16)  [unwired: 1 in]
        n153 = property on="Resolution" class="Ring (strict)"() -> ("Strings []"=w382:string[])  [unwired: 2 in, 2 out]
        n154 = call "PDCConvertResolution.vi"("ResValue"=w381, "ResStrings"=w382) -> ("Height"=w378:u32, "Width"=w379:u32)  [unwired: 8 in]
        n155 = Bundle By Name(cluster=w377, "Width"=w379, "Height"=w378) -> (w380:cluster{"Width":u32, "Height":u32})
        n156 = To Variant(anything=w380) -> (Variant=w383:variant)
        n157 = call "EnqueueMessage.vi"("error in (no error)"=w376, "MessageData"=w383, "Message"="SetResolution", "MessageQueue"=w386) -> ("error out"=w375:errorcluster)  [unwired: 6 in, 1 out]
      }
      event Value Change {
        n158 = event-data() -> ("NewVal"=w388:u16)  [unwired: 1 in]
        n159 = property on="Record Rate" class="Ring (strict)"() -> ("Strings []"=w389:string[])  [unwired: 2 in, 2 out]
        n160 = call "PDCConvertRecRate.vi"("RecRateValue"=w388, "RecRateList"=w389) -> ("RecRate"=w387:u32)  [unwired: 9 in]
        n161 = To Variant(anything=w387) -> (Variant=w390:variant)
        n162 = call "EnqueueMessage.vi"("error in (no error)"=w394, "MessageData"=w390, "Message"="SetRecordRate", "MessageQueue"=w395) -> ("error out"=w393:errorcluster)  [unwired: 6 in, 1 out]
      }
      event Value Change {
        n163 = event-data() -> ("NewVal"=w397:u16)  [unwired: 1 in]
        n164 = property on="Shutter Speed" class="Ring (strict)"() -> ("Strings []"=w398:string[])  [unwired: 2 in, 2 out]
        n165 = call "PDCConvertShutter.vi"("ShutterValue"=w397, "ShutterList"=w398) -> ("ShutterSpeed"=w396:u32)  [unwired: 9 in]
        n166 = To Variant(anything=w396) -> (Variant=w399:variant)
        n167 = call "EnqueueMessage.vi"("error in (no error)"=w403, "MessageData"=w399, "Message"="SetShutterSpeed", "MessageQueue"=w404) -> ("error out"=w402:errorcluster)  [unwired: 6 in, 1 out]
      }
      event Value Change {
        n168 = event-data() -> ("NewVal"=w407:u16)  [unwired: 1 in]
        n169 = property on="Trigger Mode" class="Ring (strict)"() -> ("Strings []"=w408:string[])  [unwired: 2 in, 2 out]
        n170 = call "PDCConvertTrigg.vi"("TriggerValue"=w407, "TriggerStrings"=w408) -> ("TriggerMode"=w406:u32)  [unwired: 9 in]
        n171 = To Variant(anything=w406) -> (Variant=w409:variant)
        n172 = call "EnqueueMessage.vi"("error in (no error)"=w412, "MessageData"=w409, "Message"="SetTriggerMode", "MessageQueue"=w413) -> ("error out"=w405:errorcluster)  [unwired: 6 in, 1 out]
      }
      event Value Change {
        n173 = event-data() -> ("NewVal"=w415:T8)  [unwired: 1 in]
        n174 = To Variant(anything=w415) -> (Variant=w416:variant)
        n175 = call "EnqueueMessage.vi"("error in (no error)"=w419, "MessageData"=w416, "Message"="SetStatus", "MessageQueue"=w420) -> ("error out"=w414:errorcluster)  [unwired: 6 in, 1 out]
      }
      event "Record": Value Change {
        n176 = event-data() -> ()  [unwired: 1 in, 1 out]
        n177 = property on="Display" class="Enum (strict)"(error in=w423, "DisabledEnum"=T15."Disabled and Grayed Out" ("Disabled")) -> (error out=w422:errorcluster)  [unwired: 1 in, 1 out]
        n178 = property on="PDCRecordStatus" class="Enum (strict)"(error in=w422) -> (error out=w426:errorcluster, "Value"=w424:T2)  [unwired: 1 in, 1 out]
        n179 = To Variant(anything=w424) -> (Variant=w425:variant)
        n180 = call "EnqueueMessage.vi"("error in (no error)"=w426, "MessageData"=w425, "Message"="Record", "MessageQueue"=w428) -> ("error out"=w429:errorcluster)  [unwired: 6 in, 1 out]
      }
      event "RecCancel": Value Change {
        n181 = event-data() -> ()  [unwired: 1 in, 1 out]
        n182 = property on="Display" class="Enum (strict)"(error in=w436, "DisabledEnum"=T15."Enabled" ("Disabled")) -> (error out=w434:errorcluster)  [unwired: 1 in, 1 out]
        n183 = call "EnqueueMessage.vi"("error in (no error)"=w434, "Message"="RecStop", "MessageQueue"=w438) -> ("error out"=w433:errorcluster)  [unwired: 7 in, 1 out]
        n184 = property on="RecCancel" class="Bool (strict)"(error in=w433, "Value"=FALSE ("RecCancel")) -> (error out=w432:errorcluster)  [unwired: 1 in, 1 out]
      }
      event "CamTab": Value Change {
        n185 = event-data() -> ()  [unwired: 1 in, 1 out]
        n186 = case shown="\"CamSAVE\"" "CamTab" {
          tunnel: w442 -> [w445 w451]
          tunnel: [w447 w449] -> w441
          frame "CamLIVE", Default {
            n187 = property on="PlayFrames" class="Bool (strict)"(error in=w445, "Value"=FALSE ("CamPlay")) -> (error out=w446:errorcluster)  [unwired: 1 in, 1 out]
            n188 = property on="Display" class="Enum (strict)"(error in=w446, "Val(Sgnl)"=PDCDisplay."Live" ("Value (Signaling)")) -> (error out=w447:errorcluster)  [unwired: 1 in, 1 out]
          }
          frame "CamSAVE" {
            n189 = property on="Display" class="Enum (strict)"(error in=w451, "Val(Sgnl)"=PDCDisplay."Memory" ("Value (Signaling)")) -> (error out=w449:errorcluster)  [unwired: 1 in, 1 out]
          }
        }
      }
      event Value Change {
        n190 = event-data() -> ("NewVal"=w453:i32)  [unwired: 1 in]
        n191 = property on="Current Frame" class="DigNum (strict)"(error in=w455, "Val(Sgnl)"=w453) -> (error out=w452:errorcluster)  [unwired: 1 in, 1 out]
      }
      event Value Change {
        n192 = event-data() -> ("OldVal"=w458:i32, "NewVal"=w460:i32)  [unwired: 1 in]
        n193 = property on="End Frame" class="DigNum (strict)"() -> ("Value"=w462:i32)  [unwired: 2 in, 2 out]
        n194 = Less?(x=w460, y=w462) -> (x < y?=w461:bool)
        n195 = case shown="True" w461 {
          tunnel: w460 -> [_ w466]
          tunnel: [w465 w474] -> w459
          tunnel: w456 -> [w465 w471]
          tunnel: w458 -> [w464 _]
          tunnel: w457 -> [_ w469]
          frame False {
            n196 = property on="Start Frame" class="DigNum (strict)"("Value"=w464) -> ()  [unwired: 2 in, 2 out]
          }
          frame True {
            n197 = To Variant(anything=w466) -> (Variant=w467:variant)
            n198 = call "EnqueueMessage.vi"("error in (no error)"=w471, "MessageData"=w467, "Message"="UpdateStartFrame", "MessageQueue"=w469) -> ("error out"=w470:errorcluster)  [unwired: 6 in, 1 out]
            n199 = property on="Frames-Slide" class="Slide (strict)"() -> ("Value"=w478:i32)  [unwired: 2 in, 2 out]
            n200 = Greater?(x=w466, y=w478) -> (0:w479:bool)
            n201 = Select(t=w466, s=w479, f=w478) -> (s? t:f=w477:i32)
            n202 = property on="Frames-Slide" class="Slide (strict)"("Scale.Minimum"=w466, "Value"=w477) -> (error out=w476:errorcluster)  [unwired: 2 in, 1 out]
            n203 = property on="Current Frame" class="DigNum (strict)"(error in=w470, "Val(Sgnl)"=w477) -> (error out=w475:errorcluster)  [unwired: 1 in, 1 out]
            n204 = Merge Errors(w476, w475) -> (w473:errorcluster)
            n205 = property on="PlayFrames" class="Bool (strict)"(error in=w473, "Val(Sgnl)"=FALSE ("Value (Signaling)")) -> (error out=w474:errorcluster)  [unwired: 1 in, 1 out]
          }
        }
      }
      event Value Change {
        n206 = event-data() -> ("OldVal"=w482:i32, "NewVal"=w484:i32)  [unwired: 1 in]
        n207 = property on="Start Frame" class="DigNum (strict)"() -> ("Value"=w486:i32)  [unwired: 2 in, 2 out]
        n208 = Greater?(x=w484, y=w486) -> (0:w485:bool)
        n209 = case shown="True" w485 {
          tunnel: w484 -> [_ w490]
          tunnel: [w489 w498] -> w483
          tunnel: w480 -> [w489 w495]
          tunnel: w482 -> [w488 _]
          tunnel: w481 -> [_ w493]
          frame False {
            n210 = property on="End Frame" class="DigNum (strict)"("Value"=w488) -> ()  [unwired: 2 in, 2 out]
          }
          frame True {
            n211 = To Variant(anything=w490) -> (Variant=w491:variant)
            n212 = call "EnqueueMessage.vi"("error in (no error)"=w495, "MessageData"=w491, "Message"="UpdateEndFrame", "MessageQueue"=w493) -> ("error out"=w494:errorcluster)  [unwired: 6 in, 1 out]
            n213 = property on="Frames-Slide" class="Slide (strict)"() -> ("Value"=w502:i32)  [unwired: 2 in, 2 out]
            n214 = Less?(x=w490, y=w502) -> (x < y?=w503:bool)
            n215 = Select(t=w490, s=w503, f=w502) -> (s? t:f=w501:i32)
            n216 = property on="Frames-Slide" class="Slide (strict)"("Scale.Maximum"=w490, "Value"=w501) -> (error out=w500:errorcluster)  [unwired: 2 in, 1 out]
            n217 = property on="Current Frame" class="DigNum (strict)"(error in=w494, "Val(Sgnl)"=w501) -> (error out=w499:errorcluster)  [unwired: 1 in, 1 out]
            n218 = Merge Errors(w500, w499) -> (w497:errorcluster)
            n219 = property on="PlayFrames" class="Bool (strict)"(error in=w497, "Val(Sgnl)"=FALSE ("Value (Signaling)")) -> (error out=w498:errorcluster)  [unwired: 1 in, 1 out]
          }
        }
      }
      event Value Change {
        n220 = event-data() -> ("NewVal"=w505:i32)  [unwired: 1 in]
        n221 = property on="End Frame" class="DigNum (strict)"() -> ("Value"=w510:i32)  [unwired: 2 in, 2 out]
        n222 = property on="Start Frame" class="DigNum (strict)"() -> ("Value"=w508:i32)  [unwired: 2 in, 2 out]
        n223 = In Range and Coerce(upper limit=w510, x=w505, lower limit=w508) -> (In Range?=w509:bool)  [unwired: 1 out]
        n224 = case shown="True" w509 {
          tunnel: w508 -> [w515 _]
          tunnel: w505 -> [_ w516]
          tunnel: [w515 w516] -> w504
          frame False {
          }
          frame True {
          }
        }
        n225 = property on="Frames-Slide" class="Slide (strict)"("Value"=w504) -> ()  [unwired: 2 in, 2 out]
        n226 = property on="Current Frame" class="DigNum (strict)"("Value"=w504) -> ()  [unwired: 2 in, 2 out]
        n227 = To Variant(anything=w504) -> (Variant=w511:variant)
        n228 = call "EnqueueMessage.vi"("error in (no error)"=w513, "MessageData"=w511, "Message"="UpdateCurrentFrame", "MessageQueue"=w506) -> ("error out"=w507:errorcluster)  [unwired: 6 in, 1 out]
      }
      event Value Change {
        n229 = event-data() -> ("NewVal"=w517:bool)  [unwired: 1 in]
        n230 = To Variant(anything=w517) -> (Variant=w519:variant)
        n231 = call "EnqueueMessage.vi"("error in (no error)"=w523, "MessageData"=w519, "Message"="TogglePlayFrames", "MessageQueue"=w520) -> ("error out"=w522:errorcluster)  [unwired: 6 in, 1 out]
      }
      event "PDCSaveFrames": Value Change {
        n232 = event-data() -> ()  [unwired: 1 in, 1 out]
        n233 = Unbundle By Name("PDC Save Settings") -> ("Save Folder"=w528:path, "File Name"=w527:string)
        n234 = Build Path(base path=w528, name or relative path=w527) -> (appended path=w526:path)
        n235 = Empty String/Path?(string/path=w526) -> (empty?=w525:bool)
        n236 = case shown="False" w525 {
          tunnel: w524 -> [w533 w544]
          tunnel: [w541 w544] -> w532
          tunnel: w530 -> [w540 _]
          tunnel: "PDC Save Settings" -> [w536 _]
          frame False {
            n237 = control-ref of="SaveStatus"() -> (w542:refnum<vi>)
            n238 = property on="CamTab" class="TabCtl (strict)"(error in=w533, "DisabledEnum"=2) -> (error out=w534:errorcluster)  [unwired: 1 in, 1 out]
            n239 = Bundle("PDC Save Settings"=w536, "SaveStatus"=w542) -> (w538:T19)  [unwired: 1 in]
            n240 = To Variant(anything=w538) -> (Variant=w539:variant)
            n241 = call "EnqueueMessage.vi"("error in (no error)"=w534, "MessageData"=w539, "Message"="PDCDataSave", "MessageQueue"=w540) -> ("error out"=w541:errorcluster)  [unwired: 6 in, 1 out]
          }
          frame True {
            n242 = One Button Dialog(message="File Name ERROR.\nPlease check \"Save Folder\"/\"File Name\".") -> ()  [unwired: 1 in, 1 out]
          }
        }
      }
      event "SavePDCSetup": Value Change {
        n243 = event-data() -> ()  [unwired: 1 in, 1 out]
        n244 = property on="Resolution" class="Ring (strict)"() -> ("Strings []"=w561:string[])  [unwired: 2 in, 2 out]
        n245 = property on="Record Rate" class="Ring (strict)"() -> ("Strings []"=w560:string[])  [unwired: 2 in, 2 out]
        n246 = property on="Shutter Speed" class="Ring (strict)"() -> ("Strings []"=w559:string[])  [unwired: 2 in, 2 out]
        n247 = property on="Trigger Mode" class="Ring (strict)"() -> ("Strings []"=w558:string[])  [unwired: 2 in, 2 out]
        n248 = property on="PDC Setup" class="Clust (strict)"() -> ("Value"=w546:T7)  [unwired: 2 in, 2 out]
        n249 = Bundle(cluster=T14 {"ResolutionList"=[], "RecordRateList"=[], "ShutterSpeedList"=[], "TriggerModeList"=[]} ("PDCLists"), "ResolutionList"=w561, "RecordRateList"=w560, "ShutterSpeedList"=w559, "TriggerModeList"=w558) -> (w547:T14)
        n250 = Bundle("PDCLists"=w547, "Value"=w546) -> (w545:cluster{"PDCLists":T14, "Value":T7})  [unwired: 1 in]
        n251 = call <vilib>:"Application Directory.vi"() -> ("Application Directory"=w556:path)
        n252 = call "File Dialog"("start path"=w556, "default name"="PDC_Setup", "pattern (all files)"="*.xml") -> ("selected path"=w550:path)  [unwired: 9 in, 3 out]
        n253 = Flatten To XML(anything=w545) -> (xml string=w557:string)
        n254 = call <vilib>:"Is Path and Not Empty.vi"("path"=w550) -> ("Is Path and Not Empty?"=w549:bool)  [unwired: 4 in]
        n255 = case shown="True" w549 {
          tunnel: w557 -> [_ w566]
          tunnel: w550 -> [_ w565]
          tunnel: w553 -> [w562 w564]
          tunnel: [w562 w563] -> w552
          frame False {
          }
          frame True {
            n256 = call-poly <vilib>:"Write to XML File.vi"("error in (no error)"=w564, "XML Input"=w566, "XML File Path"=w565) -> ("error out"=w563:errorcluster)  [unwired: 6 in, 2 out]
          }
        }
      }
      event "LoadPDCSetup": Value Change {
        n257 = event-data() -> ()  [unwired: 1 in, 1 out]
        n258 = call <vilib>:"Application Directory.vi"() -> ("Application Directory"=w574:path)
        n259 = call "File Dialog2"("start path"=w574, "pattern (all files)"="*.xml") -> ("selected path"=w569:path)  [unwired: 10 in, 3 out]
        n260 = call <vilib>:"Is Path and Not Empty.vi"("path"=w569) -> ("Is Path and Not Empty?"=w571:bool)  [unwired: 4 in]
        n261 = case shown="True" w571 {
          tunnel: w570 -> [w575 w586]
          tunnel: w569 -> [_ w585]
          tunnel: [w575 w579] -> w568
          tunnel: w567 -> [_ w581]
          frame False {
          }
          frame True {
            w582 = cluster{"PDCLists":T14, "Value":T7} {"PDCLists"={"ResolutionList"=[], "RecordRateList"=[], "ShutterSpeedList"=[], "TriggerModeList"=[]}, "Value"={"Color Type"=enum."MONO", "Bit Depth"=0, "Resolution"=0, "Record Rate"=0, "Shutter Speed"=0, "Trigger Mode"=0, "Display"=enum."Live"}}  # PDCLoadedSetup
            n262 = call-poly <vilib>:"Read From XML File.vi"("error in (no error)"=w586, "XML File Path"=w585) -> ("error out"=w583:errorcluster, "XML Elements"=w584:string)  [unwired: 7 in, 1 out]
            n263 = Unflatten From XML(xml string=w584, type=w582, error in (no error)=w583) -> (value=w577:cluster{"PDCLists":T14, "Value":T7}, error out=w580:errorcluster)
            n264 = To Variant(anything=w577) -> (Variant=w576:variant)
            n265 = call "EnqueueMessage.vi"("error in (no error)"=w580, "MessageData"=w576, "Message"="SetPDCSetup", "MessageQueue"=w581) -> ("error out"=w579:errorcluster)  [unwired: 6 in, 1 out]
          }
        }
      }
      event Value Change {
        n266 = event-data() -> ()  [unwired: 1 in, 1 out]
        n267 = To Variant(anything="Auto Trigger") -> (Variant=w588:variant)
        n268 = call "EnqueueMessage.vi"("error in (no error)"=w593, "MessageData"=w588, "Message"="ToggleAutoTrigger", "MessageQueue"=w590) -> ("error out"=w592:errorcluster)  [unwired: 6 in, 1 out]
      }
      event "Shading": Value Change {
        n269 = event-data() -> ()  [unwired: 1 in, 1 out]
        n270 = Two Button Dialog(message="WARNING:\nA black level correction is required (shading callibration).\nPlease cover the sensor before proceeding,\nPress 'OK' when ready.") -> (T button?=w595:bool)  [unwired: 2 in]
        n271 = case shown="True" w595 {
          tunnel: w599 -> [w600 w604]
          tunnel: [w600 w603] -> w598
          tunnel: w596 -> [_ w602]
          frame False {
          }
          frame True {
            n272 = call "EnqueueMessage.vi"("error in (no error)"=w604, "Message"="SetShadingMode", "MessageQueue"=w602) -> ("error out"=w603:errorcluster)  [unwired: 7 in, 1 out]
          }
        }
      }
      event "PDCStartPFV": Value Change {
        n273 = event-data() -> ()  [unwired: 1 in, 1 out]
        n274 = flat-sequence {
          tunnel: w616 -> [w623]
          tunnel: [w622] -> w612
          tunnel: w611 -> [w620]
          tunnel: [w618] -> w609
          tunnel: [w626] -> w613
          tunnel: w612 -> [w626]
          tunnel: [w624] -> w610
          tunnel: w609 -> [w624]
          tunnel: w613 -> [w634]
          tunnel: [w633] -> w608
          tunnel: [w627] -> w606
          tunnel: w610 -> [w627]
          tunnel: w608 -> [w637]
          tunnel: [w637] -> w607
          tunnel: w606 -> [w636]
          tunnel: [w636] -> w605
          tunnel: [w640] -> w615
          tunnel: w607 -> [w641]
          tunnel: w605 -> [w639]
          frame #0 {
            n275 = property class="VI"("FP.State"=3) -> ()  [unwired: 2 in, 2 out]
            n276 = call "EnqueueMessage.vi"("Priority Message? (F)"=TRUE, "error in (no error)"=w623, "Message"="PDCPause", "MessageQueue"=w620) -> ("error out"=w622:errorcluster, "dupMessageQueue"=w618:refnum<queue>)  [unwired: 6 in]
          }
          frame #1 {
            n277 = Wait (ms)(milliseconds to wait=u32 500) -> ()  [unwired: 1 out]
          }
          frame #2 {
            n278 = Path To String(path="Path of PFV.exe") -> (string=w630:string)
            n279 = Concatenate Strings("\"", w630, "\"") -> (w628:string)
            n280 = call <vilib>:"System Exec.vi"("error in (no error)"=w634, "command line"=w628) -> ("error out"=w633:errorcluster)  [unwired: 6 in, 3 out]
          }
          frame #3 {
            n281 = Wait (ms)(milliseconds to wait=u32 500) -> ()  [unwired: 1 out]
          }
          frame #4 {
            n282 = property class="VI"("FP.State"=1) -> ()  [unwired: 2 in, 2 out]
            n283 = call "EnqueueMessage.vi"("error in (no error)"=w641, "Message"="ReInitialize", "MessageQueue"=w639) -> ("error out"=w640:errorcluster)  [unwired: 7 in, 1 out]
          }
        }
      }
      event "Run Calibration": Value Change {
        n284 = event-data() -> ()  [unwired: 1 in, 1 out]
        n285 = flat-sequence {
          tunnel: w645 -> [w661]
          tunnel: [w660] -> w654
          tunnel: w644 -> [w658]
          tunnel: [w656] -> w653
          tunnel: [w664] -> w652
          tunnel: w654 -> [w664]
          tunnel: [w662] -> w651
          tunnel: w653 -> [w662]
          tunnel: w652 -> [w671]
          tunnel: [w670] -> w650
          tunnel: [w669] -> w649
          tunnel: w651 -> [w669]
          tunnel: w650 -> [w674]
          tunnel: [w674] -> w648
          tunnel: w649 -> [w673]
          tunnel: [w673] -> w647
          tunnel: [w677] -> w646
          tunnel: w648 -> [w678]
          tunnel: w647 -> [w676]
          frame #0 {
            n286 = property class="VI"("FP.State"=3) -> ()  [unwired: 2 in, 2 out]
            n287 = call "EnqueueMessage.vi"("Priority Message? (F)"=TRUE, "error in (no error)"=w661, "Message"="Pause", "MessageQueue"=w658) -> ("error out"=w660:errorcluster, "dupMessageQueue"=w656:refnum<queue>)  [unwired: 6 in]
          }
          frame #1 {
            n288 = Wait (ms)(milliseconds to wait=u32 500) -> ()  [unwired: 1 out]
          }
          frame #2 {
            n289 = call <vilib>:"Application Directory.vi"() -> ("Application Directory"=w666:path)
            n290 = Build Path(base path=w666, name or relative path="Calibration.exe") -> (appended path=w668:path)
            n291 = Path To String(path=w668) -> (string=w665:string)
            n292 = call <vilib>:"System Exec.vi"("error in (no error)"=w671, "command line"=w665) -> ("error out"=w670:errorcluster)  [unwired: 6 in, 3 out]
          }
          frame #3 {
            n293 = Wait (ms)(milliseconds to wait=u32 500) -> ()  [unwired: 1 out]
          }
          frame #4 {
            n294 = property class="VI"("FP.State"=1) -> ()  [unwired: 2 in, 2 out]
            n295 = call "EnqueueMessage.vi"("error in (no error)"=w678, "Message"="ReInitialize", "MessageQueue"=w676) -> ("error out"=w677:errorcluster)  [unwired: 7 in, 1 out]
          }
        }
      }
      event "ConfigureCls": Value Change {
        n296 = event-data() -> ()  [unwired: 1 in, 6 out]
        n297 = call "EnqueueMessage.vi"("error in (no error)"=w682, "Message"="ConfigureCls", "MessageQueue"=w684) -> ("error out"=w681:errorcluster)  [unwired: 7 in, 1 out]
      }
    }
    n298 = call "ErrorModule.vi"("Error In"=w230, "CommunicationRefs"=w229) -> ("Error Out"=w231:errorcluster)  [unwired: 9 in]
  }
  n299 = Unregister For Events(event registration refnum=w33) -> (error out=w28:errorcluster)  [unwired: 1 in]
  n300 = Merge Errors(w29, w28, w22, w27, w26, w25, w24, w15, w14, w8, w7) -> (w32:errorcluster)
  n301 = call "ClearAll.vi"("Error In"=w32, "CommunicationRefs"=w1) -> ("error out"=w35:errorcluster)  [unwired: 9 in]
  n302 = call <vilib>:"Simple Error Handler.vi"("error in (no error)"=w35) -> ()  [unwired: 4 in, 5 out]
